vi "Hysteresis_max-LAPTOP-A1ILEVN9.vi"(0 "input(+)":dbl, 2 "type":enum16{"percentage", "level"}(ring), 5 "input (-)":dbl, 7 "H":dbl=22.0 format="%#_13g", 9 "Max":dbl=26.0 format="%#_13g", 11 "error in":errorcluster) -> (8 "Deviation":bool, 15 "error out":errorcluster)   [LabVIEW 2022 SP3]
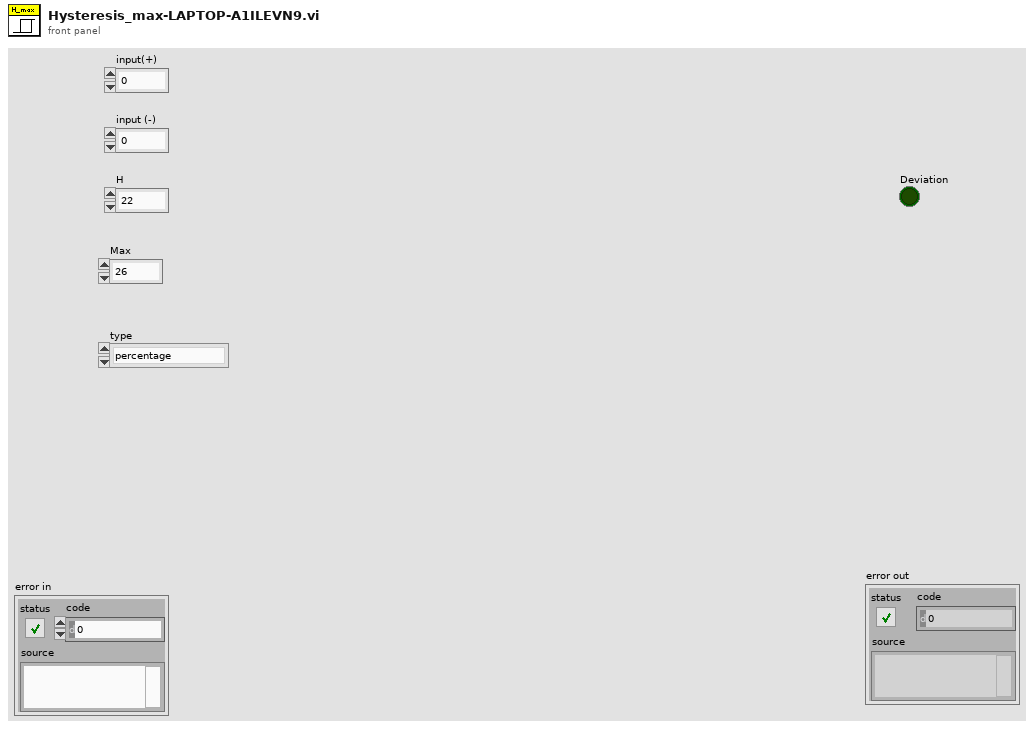
[diagram p1: front panel]
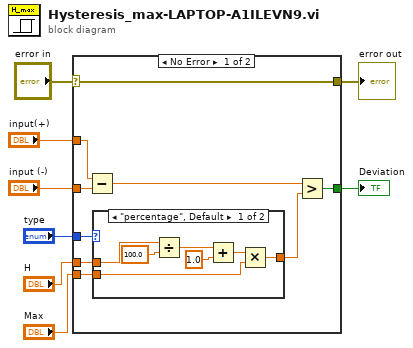
[diagram p0: block diagram]
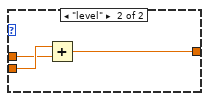
[diagram p2: hidden frame]
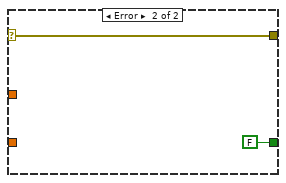
[diagram p3: hidden frame]
diagram:
  n1 = case shown="No Error" "error in" {
    selector: "error in" -> [w16 w29]
    tunnel: [w16 w29] -> w7
    tunnel: "input(+)" -> [w15 _]
    tunnel: "input (-)" -> [w14 _]
    tunnel: "H" -> [w10 _]
    tunnel: "Max" -> [w11 _]
    tunnel: [w13 FALSE] -> w2
    tunnel: "type" -> [w12 _]
    frame No Error {
      n2 = Subtract(x=w15, y=w14) -> (x-y=w17:dbl)
      n3 = case shown="\"percentage\", Default" w12 {
        tunnel: w11 -> [w22 w26]
        tunnel: w10 -> [w19 w25]
        tunnel: [w18 w27] -> w9
        frame "percentage", Default {
          n4 = Divide(x=w19, y=100.0) -> (x/y=w24:dbl)
          n5 = Add(x=w24, y=1.0) -> (x+y=w23:dbl)
          n6 = Multiply(x=w23, y=w22) -> (x*y=w18:dbl)
        }
        frame "level" {
          n7 = Add(x=w26, y=w25) -> (x+y=w27:dbl)
        }
      }
      n8 = Greater?(x=w17, y=w9) -> (0:w13:bool)
    }
    frame Error {
    }
  }
  "error out" <- w7
  "Deviation" <- w2
